vi "吸声系数as计算.vi"(10 "试件吸声量AT":dbl[](array[numeric])) -> (2 "吸声系数as":dbl[](array[numeric]))   [LabVIEW 2020]
uses:
  setup/support/rev_setup.lvlib
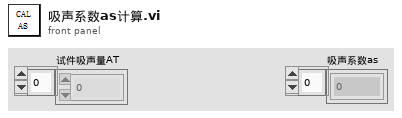
[diagram p1: front panel]
types:
  T1 = typedef "rev_setup.lvlib/EMdata.ctl" = cluster{"大气压力(kPa)":dbl, "大气压力(kPa) 2":dbl, "相对湿度(%)":dbl, "相对湿度(%)2":dbl, "大气温度(℃)":dbl, "大气温度(℃)2":dbl, "声速(m/s)":dbl, "声速(kPa)2":dbl, "混响室容积(立方米) ":dbl, "试件面积(平方米)，S":dbl, "分立吸声体个数，n":dbl}
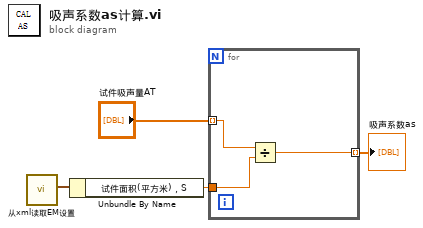
[diagram p0: block diagram]
diagram:
  n1 = call "从xml读取EM设置.vi"() -> ("EM data"=w4:T1)  [unwired: 11 in]
  n2 = Unbundle By Name(w4) -> ("试件面积(平方米)，S"=w3:dbl)
  n3 = for {
    tunnel: "试件吸声量AT" -> [w7] mode=indexing
    tunnel: w3 -> [w6]
    tunnel: [w5] -> w2 mode=indexing
    n4 = Divide(x=w7, y=w6) -> (x/y=w5:dbl)
  }
  "吸声系数as" <- w2
